vi "Getproperty_id.vi"(8 "error in (no error)":errorcluster, 11 "OneOfTemplate in":refnum<class "nixnet_grpc_GetSubPropertyRequest_subproperty_id_enum.lvclass">) -> (0 "error out":errorcluster, 2 "Get_Val":T1, 3 "OneOfTemplate out":refnum<class "nixnet_grpc_GetSubPropertyRequest_subproperty_id_enum.lvclass">)   [LabVIEW 2019, in "grpc-xnet_client.lvlib" / "nixnet_grpc_GetSubPropertyRequest_subproperty_id_enum.lvclass"]
uses:
  nixnet_grpc_GetSubPropertyRequest_subproperty_id_enum.lvclass
  nixnet_grpc_SubProperty.ctl
  nixnet_grpc_GetSubPropertyRequest_subproperty_id_enum.lvclass/nixnet_grpc_GetSubPropertyRequest_subproperty_id_enum.ctl
  grpc-xnet_client.lvlib
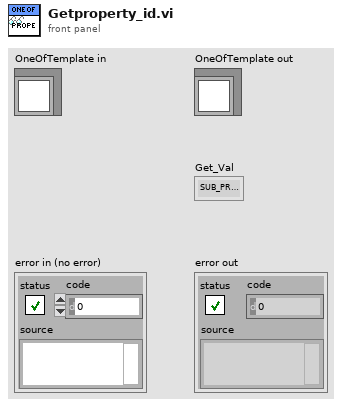
[diagram p1: front panel]
types:
  T1 = typedef "grpc-xnet_client.lvlib/nixnet_grpc_SubProperty.ctl" = enum32{"SUB_PROPERTY_UNSPECIFIED", "SUB_PROPERTY_SESSION_SUB_CAN_START_TIME_OFF", "SUB_PROPERTY_SESSION_SUB_CAN_TX_TIME", "SUB_PROPERTY_SESSION_SUB_LIN_TX_N_CORRUPTED_CHKSUMS", "SUB_PROPERTY_SESSION_SUB_OUTPUT_QUEUE_UPDATE_FREQ", "SUB_PROPERTY_SESSION_SUB_J1939_ADDR_FILTER", "SUB_PROPERTY_SESSION_SUB_SKIP_N_CYCLIC_FRAMES"}
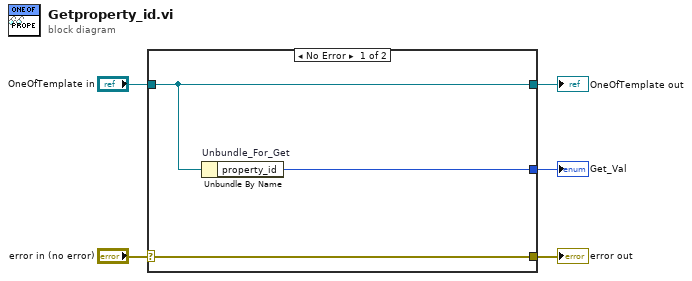
[diagram p0: block diagram]
diagram:
  n1 = case shown="No Error" "error in (no error)" {
    selector: "error in (no error)" -> [w8 w9]
    tunnel: [w8 w9] -> w4
    tunnel: [w7 w10] -> w2
    tunnel: "OneOfTemplate in" -> [w7 w10]
    tunnel: [w6 _] -> w1
    frame No Error {
      n2 = Unbundle By Name "Unbundle_For_Get"(w7) -> ("property_id"=w6:T1)
    }
    frame Error {
    }
  }
  "error out" <- w4
  "OneOfTemplate out" <- w2
  "Get_Val" <- w1
